vi "ReadSystemDefinitionOverrideFile.vi"(8 "error in (no error)":errorcluster, 11 "configuration file path":path) -> (0 "error out":errorcluster, 3 "override items":T1(array[cluster]))   [LabVIEW 2015, in "VeriStandTestCase.lvclass"]
uses:
  VeriStandTestCase.lvclass
  OverrideItem.ctl
  <vilib>/Utility/config.llb/Read Key (String).vi
  <vilib>/Utility/config.llb/NI_LVConfig.lvlib
panel:
  in  "override item":T2
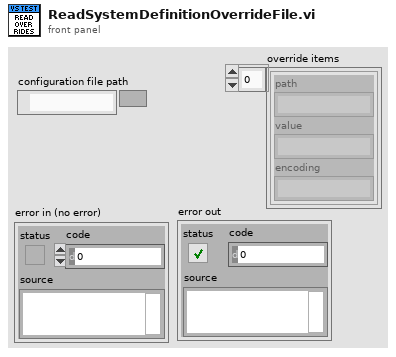
[diagram p1: front panel]
types:
  T1 = cluster{"path":string, "value":string, "encoding":string}[]
  T2 = typedef "VeriStandTestCase.lvclass/OverrideItem.ctl" = cluster{"path":string, "value":string, "encoding":string}
  T3 = typedef "NI_LVConfig.lvlib/Config Data RefNum.ctl" = refnum<k1>
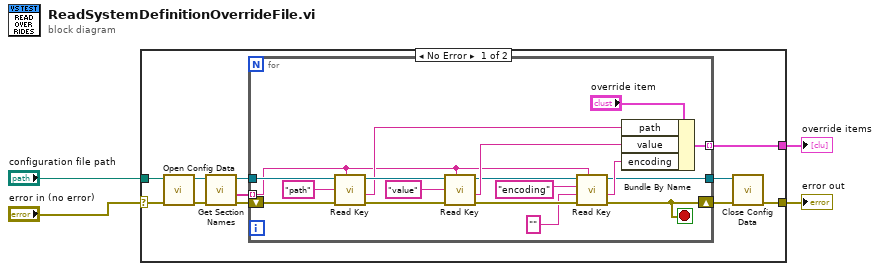
[diagram p0: block diagram]
diagram:
  n1 = case shown="No Error" "error in (no error)" {
    selector: "error in (no error)" -> [w6 w34]
    tunnel: [w15 w34] -> w4
    tunnel: "configuration file path" -> [w14 _]
    tunnel: [w5 _] -> w1
    frame No Error {
      n2 = call <vilib>:"Open Config Data.vi"("error in (no error)"=w6, "configuration file path"=w14) -> ("error out"=w7:errorcluster, "refnum"=w8:T3)  [unwired: 7 in, 1 out]
      n3 = call <vilib>:"Get Section Names.vi"("error in (no error)"=w7, "refnum"=w8) -> ("error out"=w11:errorcluster, "section names"=w9:string[], "refnum out"=w10:T3)  [unwired: 7 in]
      n4 = for {
        tunnel: w9 -> [w19] mode=indexing
        tunnel: w10 -> [w33]
        tunnel: [w16] -> w12
        tunnel: [w20] -> w5 mode=indexing
        shift-right: [w23] -> w13
        shift-left: w11 -> [w32]
        stop <- w23 stop-if-true
        n5 = call-poly <vilib>:"Read Key.vi"("section"=w19, "error in (no error)"=w32, "key"="path", "refnum"=w33) -> ("error out"=w30:errorcluster, "value"=w26:string, "refnum out"=w29:T3)  [unwired: 4 in, 1 out]
        n6 = call-poly <vilib>:"Read Key.vi"("section"=w19, "error in (no error)"=w30, "key"="value", "refnum"=w29) -> ("error out"=w24:errorcluster, "value"=w28:string, "refnum out"=w17:T3)  [unwired: 4 in, 1 out]
        n7 = call-poly <vilib>:"Read Key.vi"("section"=w19, "error in (no error)"=w24, "default value"="", "key"="encoding", "refnum"=w17) -> ("error out"=w23:errorcluster, "value"=w18:string, "refnum out"=w16:T3)  [unwired: 3 in, 1 out]
        n8 = Bundle By Name(cluster="override item", "path"=w26, "value"=w28, "encoding"=w18) -> (w20:T2)
      }
      n9 = call <vilib>:"Close Config Data.vi"("error in (no error)"=w13, "refnum"=w12) -> ("error out"=w15:errorcluster)  [unwired: 8 in, 1 out]
    }
    frame Error {
    }
  }
  "error out" <- w4
  "override items" <- w1
